vi "Swap I16s of U64.vi"(7 "Number":u64) -> (8 "swapped number":u64)   [LabVIEW 2012]
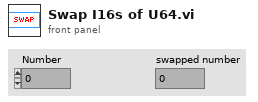
[diagram p1: front panel]
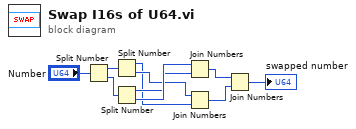
[diagram p0: block diagram]
diagram:
  n1 = Split Number(x="Number") -> (hi(x)=w9:u32, lo(x)=w10:u32)
  n2 = Split Number(x=w9) -> (hi(x)=w3:u16, lo(x)=w4:u16)
  n3 = Split Number(x=w10) -> (hi(x)=w5:u16, lo(x)=w6:u16)
  n4 = Join Numbers(hi=w6, lo=w5) -> ((hi.lo)=w8:u32)
  n5 = Join Numbers(hi=w4, lo=w3) -> ((hi.lo)=w7:u32)
  n6 = Join Numbers(hi=w8, lo=w7) -> ((hi.lo)=→"swapped number":u64)
